vi "ex3_moje.vi"() -> ()   [LabVIEW 2022 SP3]
panel:
  out "data":bool[][](array[boolean])
  in  "Boolean array":bool[][](array[boolean])
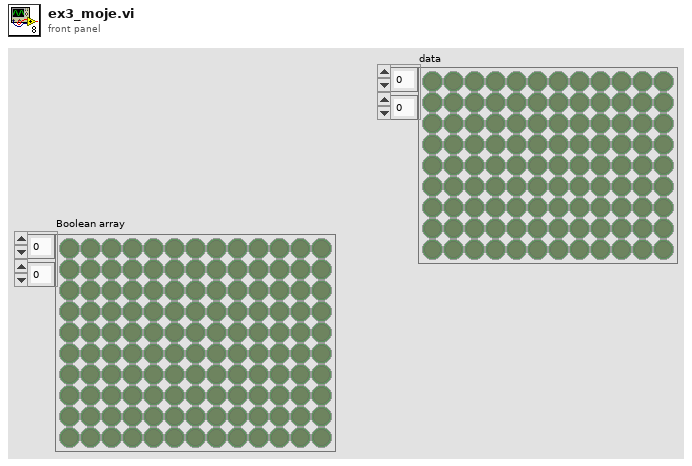
[diagram p1: front panel]
types:
  T1 = enum16{"open", "replace", "create", "open or create", "replace or create", "replace or create with confirmation"}
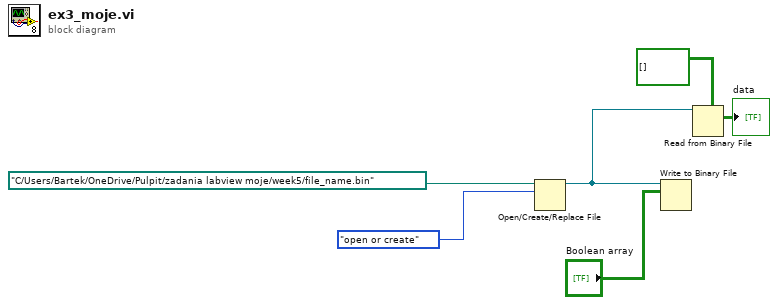
[diagram p0: block diagram]
diagram:
  n1 = Open/Create/Replace File(file path (use dialog)=path "C:/Users/Bartek/OneDrive/Pulpit/zadania labview moje/week5/file_name.bin", operation (0:open)=T1."open or create") -> (refnum out=w3:refnum<file>)  [unwired: 4 in, 2 out]
  n2 = Write to Binary File(file (use dialog)=w3, data="Boolean array") -> ()  [unwired: 4 in, 3 out]
  n3 = Read from Binary File(5:bool[][] [] ("Array"), 11:w3) -> (2:→"data":bool[][])  [unwired: 4 in, 3 out]
